vi "Extract Inner Message.vi"(7 "Copy":bool caption="Copy data instead of extracting", 8 "error in (no error)":errorcluster, 11 "Message in":refnum<class "MSG.lvclass">) -> (0 "error out":errorcluster, 1 "Inner Message":refnum<class "MSG.lvclass">, 2 "Outer Envelope Label":string, 3 "Message (outer envelope) out":refnum<class "MSG.lvclass">)   [LabVIEW 2011, in "Messenging.lvlib" / "MSG.lvclass"]
uses:
  MSG.lvclass
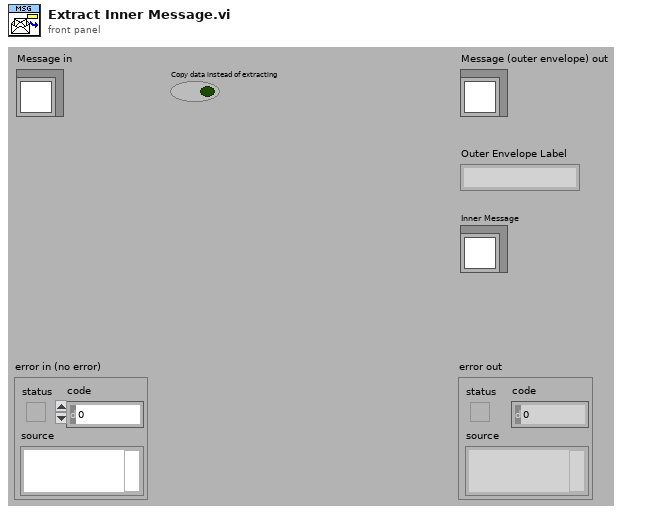
[diagram p1: front panel]
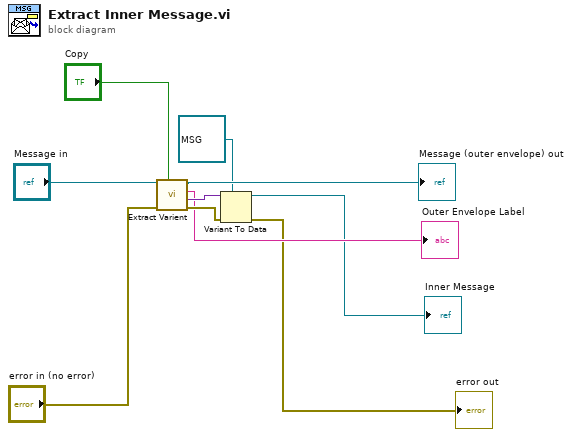
[diagram p0: block diagram]
diagram:
  n1 = call-dynamic "Extract Varient.vi"("Copy"="Copy", "error in (no error)"="error in (no error)", "Message"="Message in") -> ("error out"=w9:errorcluster, "Varient"=w10:variant, "Label"=→"Outer Envelope Label":string, "Message"=→"Message (outer envelope) out":refnum<class "MSG.lvclass">)  [unwired: 5 out]
  n2 = Variant To Data(error in=w9, type=refnum<class "MSG.lvclass"> refnum ("Messenging.lvlib:Interprocess Message"), Variant=w10) -> (data=→"Inner Message":refnum<class "MSG.lvclass">, error out=→"error out":errorcluster)
